vi "Write Duty Cycle.vi"(8 "error in (no error)":errorcluster, 10 "DC":dbl, 11 "Update Laser rate and DC in":refnum<class "Update Laser rate and DC.lvclass">) -> (0 "error out":errorcluster, 3 "Update Laser rate and DC out":refnum<class "Update Laser rate and DC.lvclass">)   [LabVIEW 2014, in "eCRDS Library.lvlib" / "Update Laser rate and DC.lvclass"]
uses:
  Update Laser rate and DC.lvclass
  Update Laser rate and DC.lvclass/Update Laser rate and DC.ctl
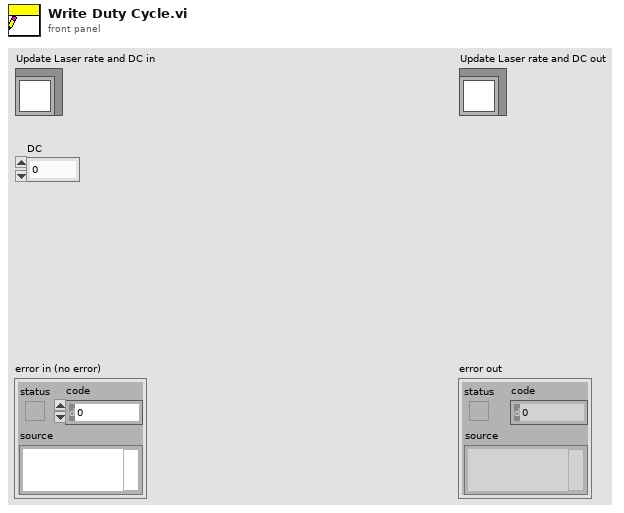
[diagram p1: front panel]
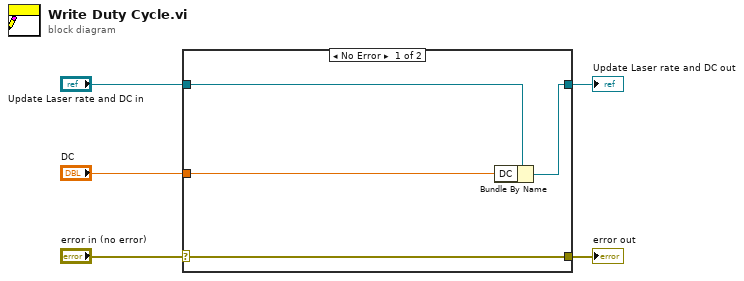
[diagram p0: block diagram]
diagram:
  n1 = case shown="No Error" "error in (no error)" {
    selector: "error in (no error)" -> [w9 w10]
    tunnel: [w9 w10] -> w4
    tunnel: [w7 w11] -> w2
    tunnel: "Update Laser rate and DC in" -> [w8 w11]
    tunnel: "DC" -> [w6 _]
    frame No Error {
      n2 = Bundle By Name(cluster=w8, "DC"=w6) -> (w7:refnum<class "Update Laser rate and DC.lvclass">)
    }
    frame Error {
    }
  }
  "error out" <- w4
  "Update Laser rate and DC out" <- w2
